vi "公式写入.vi"(5 "公式 2":cluster{"X^2":dbl, "X":dbl, "b":dbl}, 6 "公式切换阈值滴定数(0-9999)":u16, 7 "公式":cluster{"X^2":dbl, "X":dbl, "b":dbl}, 8 "Error in":errorcluster caption="Error in (no error)", 9 "量程选择":enum16{"低量程", "高量程"}(ring), 11 "模型":enum32{"线性", "多项式", "折线"}(ring)) -> (0 "error out":errorcluster)   [LabVIEW 2016, in "斯坦道CODMn.lvlib"]
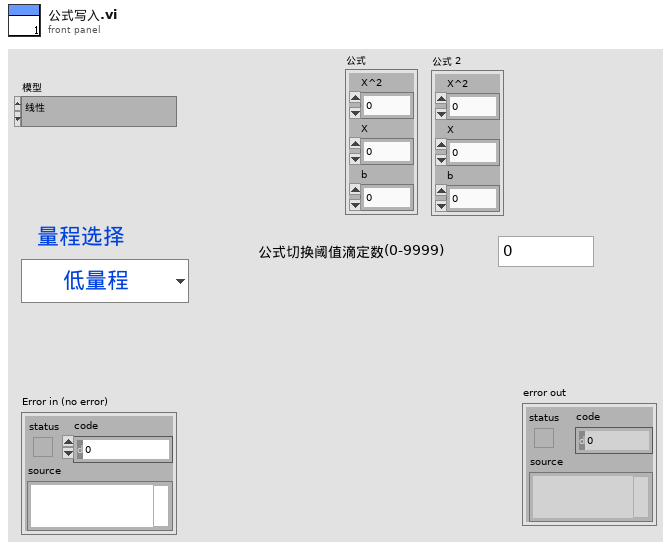
[diagram p1: front panel]
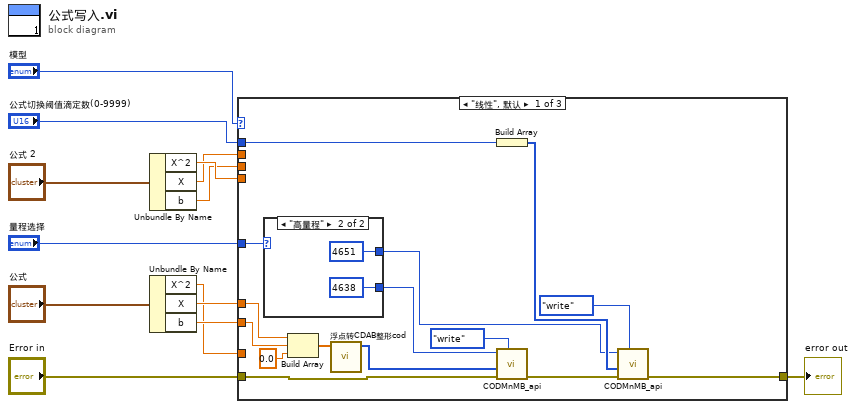
[diagram p0: block diagram]
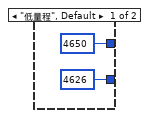
[diagram p2: hidden frame]
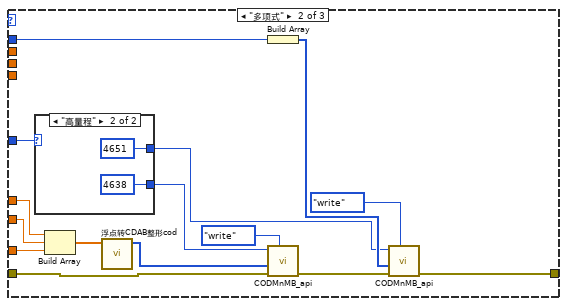
[diagram p3: hidden frame]
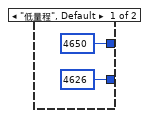
[diagram p4: hidden frame]
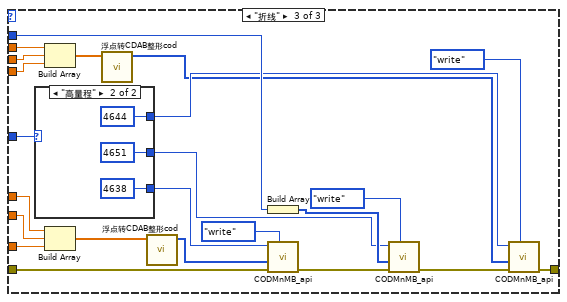
[diagram p5: hidden frame]
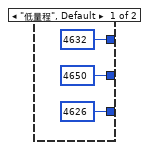
[diagram p6: hidden frame]
diagram:
  n1 = Unbundle By Name("公式 2") -> ("X^2"=w3:dbl, "X"=w2:dbl, "b"=w1:dbl)
  n2 = Unbundle By Name("公式") -> ("X^2"=w9:dbl, "X"=w10:dbl, "b"=w11:dbl)
  n3 = case shown="\"线性\", 默认" "模型" {
    tunnel: w11 -> [w26 w44 w71]
    tunnel: w10 -> [w27 w45 w72]
    tunnel: w9 -> [_ w46 w73]
    tunnel: "量程选择" -> [w24 w37 w64]
    tunnel: "Error in" -> [w21 w34 w61]
    tunnel: [w17 w33 w52] -> w6
    tunnel: "公式切换阈值滴定数(0-9999)" -> [w16 w35 w62]
    tunnel: w3 -> [_ _ w56]
    tunnel: w2 -> [_ _ w58]
    tunnel: w1 -> [_ _ w57]
    frame "线性", Default {
      n4 = case shown="\"高量程\"" w24 {
        tunnel: [u16 4626 ("starting address") u16 4638 ("starting address")] -> w22
        tunnel: [u16 4650 ("starting address") u16 4651 ("starting address")] -> w14
        frame "低量程", Default {
        }
        frame "高量程" {
        }
      }
      n5 = Build Array(w27, w26, 0.0 ("元素")) -> (w28:dbl[])
      n6 = call "浮点转CDAB整形cod.vi"("浮点数"=w28) -> ("CDAB整形输出"=w20:u16[])  [unwired: 10 in]
      n7 = Build Array(w16) -> (w15:u16[])
      n8 = call "CODMnMB_api.vi"("STEP"=enum16{"open", "read", "write", "close"}."write", "Error in"=w21, "values"=w20, "starting address"=w22) -> ("error out"=w18:errorcluster)  [unwired: 5 in, 2 out]
      n9 = call "CODMnMB_api.vi"("STEP"=enum16{"open", "read", "write", "close"}."write", "Error in"=w18, "values"=w15, "starting address"=w14) -> ("error out"=w17:errorcluster)  [unwired: 5 in, 2 out]
    }
    frame "多项式" {
      n10 = case shown="\"高量程\"" w37 {
        tunnel: [u16 4626 ("starting address") u16 4638 ("starting address")] -> w42
        tunnel: [u16 4650 ("starting address") u16 4651 ("starting address")] -> w38
        frame "低量程", Default {
        }
        frame "高量程" {
        }
      }
      n11 = Build Array(w45, w44, w46) -> (w47:dbl[])
      n12 = call "浮点转CDAB整形cod.vi"("浮点数"=w47) -> ("CDAB整形输出"=w36:u16[])  [unwired: 10 in]
      n13 = Build Array(w35) -> (w39:u16[])
      n14 = call "CODMnMB_api.vi"("STEP"=enum16{"open", "read", "write", "close"}."write", "Error in"=w34, "values"=w36, "starting address"=w42) -> ("error out"=w40:errorcluster)  [unwired: 5 in, 2 out]
      n15 = call "CODMnMB_api.vi"("STEP"=enum16{"open", "read", "write", "close"}."write", "Error in"=w40, "values"=w39, "starting address"=w38) -> ("error out"=w33:errorcluster)  [unwired: 5 in, 2 out]
    }
    frame "折线" {
      n16 = case shown="\"高量程\"" w64 {
        tunnel: [u16 4626 ("starting address") u16 4638 ("starting address")] -> w69
        tunnel: [u16 4650 ("starting address") u16 4651 ("starting address")] -> w65
        tunnel: [u16 4632 ("starting address") u16 4644 ("starting address")] -> w55
        frame "低量程", Default {
        }
        frame "高量程" {
        }
      }
      n17 = Build Array(w58, w57, w56) -> (w59:dbl[])
      n18 = Build Array(w72, w71, w73) -> (w74:dbl[])
      n19 = call "浮点转CDAB整形cod.vi"("浮点数"=w59) -> ("CDAB整形输出"=w54:u16[])  [unwired: 10 in]
      n20 = call "浮点转CDAB整形cod.vi"("浮点数"=w74) -> ("CDAB整形输出"=w63:u16[])  [unwired: 10 in]
      n21 = Build Array(w62) -> (w66:u16[])
      n22 = call "CODMnMB_api.vi"("STEP"=enum16{"open", "read", "write", "close"}."write", "Error in"=w61, "values"=w63, "starting address"=w69) -> ("error out"=w67:errorcluster)  [unwired: 5 in, 2 out]
      n23 = call "CODMnMB_api.vi"("STEP"=enum16{"open", "read", "write", "close"}."write", "Error in"=w67, "values"=w66, "starting address"=w65) -> ("error out"=w53:errorcluster)  [unwired: 5 in, 2 out]
      n24 = call "CODMnMB_api.vi"("STEP"=enum16{"open", "read", "write", "close"}."write", "Error in"=w53, "values"=w54, "starting address"=w55) -> ("error out"=w52:errorcluster)  [unwired: 5 in, 2 out]
    }
  }
  "error out" <- w6
